vi "WFDC Get Current Z Drift.vi"(0 "Ref Images":T1[](array[typedef]), 2 "Z Calibration (slope, inter)":dbl[](array[numeric]), 7 "Current Image":u16[][](array[numeric]), 11 "Error In":errorcluster) -> (8 "Z Position (µm)":dbl format="%#_10g", 15 "Error Out":errorcluster)   [LabVIEW 2020]
uses:
  <vilib>/vision/Image Controls.llb/IMAQ Image.ctl
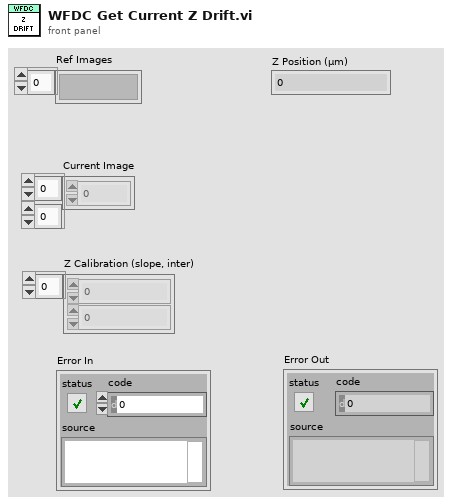
[diagram p1: front panel]
types:
  T1 = typedef "IMAQ Image.ctl" = refnum<image>
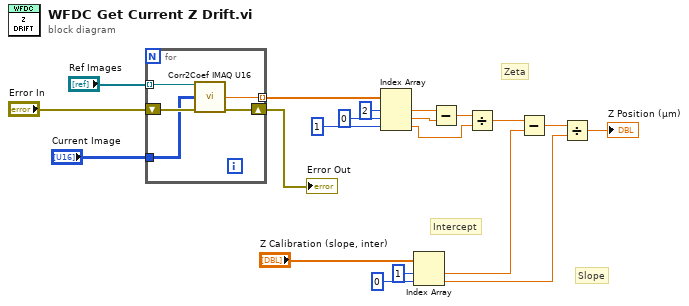
[diagram p0: block diagram]
diagram:
  # "Slope"
  # "Zeta"
  # "Intercept"
  n1 = for {
    tunnel: "Ref Images" -> [w25] mode=indexing
    shift-right: [w22] -> w1
    shift-left: "Error In" -> [w24]
    tunnel: "Current Image" -> [w23]
    tunnel: [w21] -> w8 mode=indexing
    n2 = call "Corr2Coef IMAQ U16.vi"("Image A"=w25, "Image B"=w23, "Error In"=w24) -> ("Corr Coef"=w21:dbl, "Error Out"=w22:errorcluster)  [unwired: 11 in]
  }
  "Error Out" <- w1
  n3 = Index Array(array=w8, index #1=2 ("index"), index #2=0 ("index"), index #3=1 ("index")) -> (element #1=w4:dbl, element #2=w3:dbl, element #3=w2:dbl)
  n4 = Index Array(array="Z Calibration (slope, inter)", index #1=1 ("index"), index #2=0 ("index")) -> (element #1=w14:dbl, element #2=w12:dbl)
  n5 = Subtract(x=w4, y=w3) -> (x-y=w20:dbl)
  n6 = Divide(x=w20, y=w2) -> (x/y=w15:dbl)
  n7 = Subtract(x=w15, y=w14) -> (x-y=w13:dbl)
  n8 = Divide(x=w13, y=w12) -> (x/y=→"Z Position (µm)":dbl)
